vi "Setup TestRunner Project.vi"(5 "Interactive (T)":bool=TRUE, 6 "Virtual Folder (empty: \"My Computer\")":string, 7 "Verbose (F)":bool, 8 "error in (no error)":errorcluster, 9 "Test Report":refnum<class "Test Report.lvclass">, 10 "Project Refnum":refnum<vi>, 11 "Test Runner.Project in":refnum<class "Test Runner.Project.lvclass">) -> (0 "error out":errorcluster, 3 "Test Runner.Project out":refnum<class "Test Runner.Project.lvclass">)   [LabVIEW 2013, in "Caraya.lvlib" / "Test Runner.Project.lvclass"]
uses:
  Test Runner.Project.lvclass
  Test Report/Test Report.lvclass
  Test Runner/Test Runner.lvclass/Test Runner.ctl
  Test Runner.Project.lvclass/Test Runner.Project.ctl
  Test Runner/Test Runner.lvclass
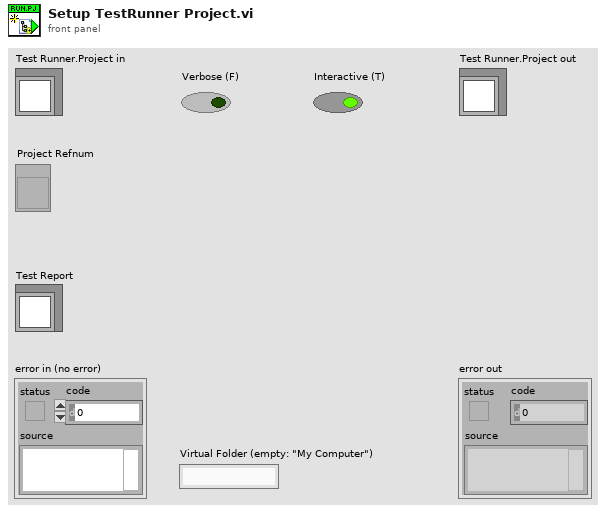
[diagram p1: front panel]
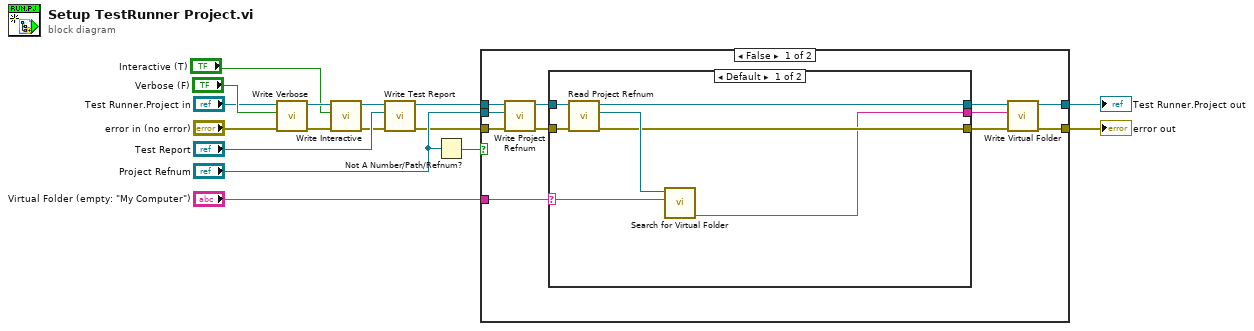
[diagram p0: block diagram]
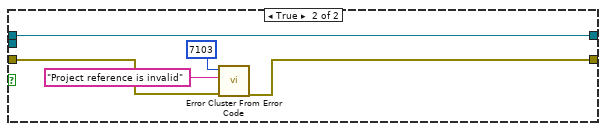
[diagram p3: hidden frame]
diagram:
  n1 = call "Write Verbose.vi"("Verbose"="Verbose (F)", "Test Runner in"="Test Runner.Project in") -> ("Test Runner out"=w5:refnum<class "Test Runner.Project.lvclass">)  [unwired: 9 in]
  n2 = call "Write Interactive.vi"("Interactive"="Interactive (T)", "Test Runner in"=w5) -> ("Test Runner out"=w2:refnum<class "Test Runner.Project.lvclass">)  [unwired: 9 in]
  n3 = call "Write Test Report.vi"("Test Report"="Test Report", "Test Runner in"=w2) -> ("Test Runner out"=w12:refnum<class "Test Runner.Project.lvclass">)  [unwired: 9 in]
  n4 = Not A Number/Path/Refnum?(number/path/refnum="Project Refnum") -> (NaN/Path/Refnum?=w10:bool)
  n5 = case shown="False" w10 {
    tunnel: w12 -> [w23 w33]
    tunnel: "error in (no error)" -> [w22 w35]
    tunnel: [w16 w33] -> w8
    tunnel: [w19 w34] -> w7
    tunnel: "Project Refnum" -> [w21 _]
    tunnel: "Virtual Folder (empty: \"My Computer\")" -> [w17 _]
    frame False {
      n6 = call "Write Project Refnum.vi"("error in (no error)"=w22, "Project Refnum"=w21, "Test Runner.Project in"=w23) -> ("error out"=w20:errorcluster, "Test Runner.Project out"=w18:refnum<class "Test Runner.Project.lvclass">)  [unwired: 7 in]
      n7 = case shown="Default" w17 {
        selector: w17 -> [w26 _]
        tunnel: w20 -> [w29 w32]
        tunnel: [w25 w32] -> w19
        tunnel: [w28 w31] -> w15
        tunnel: w18 -> [w30 w31]
        tunnel: [w24 _] -> w14
        frame Default {
          n8 = call "Read Project Refnum.vi"("error in (no error)"=w29, "Test Runner.Project in"=w30) -> ("error out"=w25:errorcluster, "Project Refnum"=w27:refnum<vi>, "Test Runner.Project out"=w28:refnum<class "Test Runner.Project.lvclass">)  [unwired: 7 in]
          n9 = call "Search for Virtual Folder.vi"("Virtual Folder"=w26, "Project Refnum"=w27) -> ("Best Match Name"=w24:string)  [unwired: 6 in, 3 out]
        }
        frame "" {
        }
      }
      n10 = call "Write Virtual Folder.vi"("Virtual Folder"=w14, "Test Runner.Project in"=w15) -> ("Test Runner.Project out"=w16:refnum<class "Test Runner.Project.lvclass">)  [unwired: 9 in]
    }
    frame True {
      n11 = call <vilib>:"Error Cluster From Error Code.vi"("error in (no error)"=w35, "error message (\"\")"="Project reference is invalid" ("error message (\"\")"), "error code (0)"=7103) -> ("error out"=w34:errorcluster)  [unwired: 6 in]
    }
  }
  "error out" <- w7
  "Test Runner.Project out" <- w8
